vi "FrameParser.vi"(0 "DataIn":u8[](array[numeric]), 1 "frameBuffer":u8[](array[numeric]), 3 "state_in":i32, 4 "dataCnt_in":i32) -> (13 "frameComplete":i32, 14 "frame_data":u8[](array[numeric]), 15 "frame_size":i32, 16 "DataOut":u8[](array[numeric]), 17 "rest":i32, 18 "state_out":i32, 19 "fdataCnt":i32)   [LabVIEW 2017]
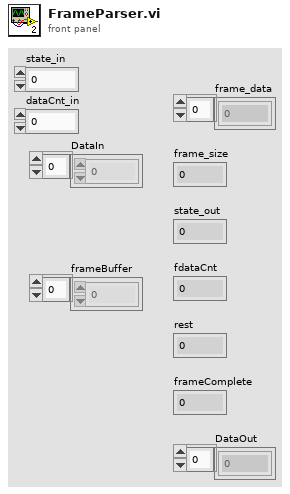
[diagram p1: front panel]
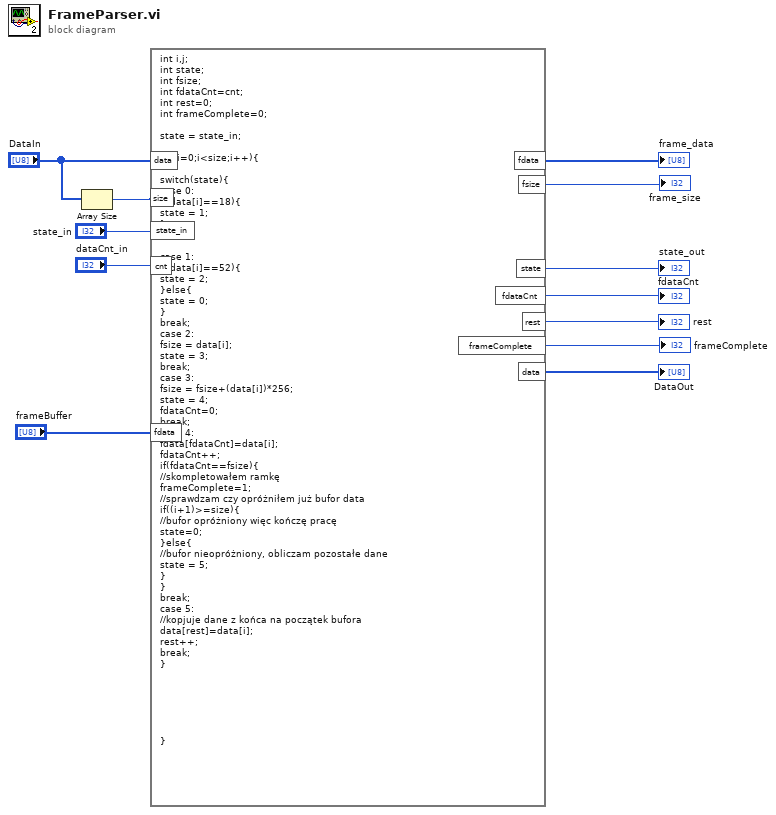
[diagram p0: block diagram]
diagram:
  n1 = Array Size(array="DataIn") -> (size(s)=w3:i32)
  n2 = formula code="int i,j;\nint state;\nint fsize;\nint fdataCnt=cnt;\nint rest=0;\nint frameComplete=0;\n\nstate = state_in;\n\nfor(i=0;i<size;i++){\n\nswitch(state){\ncase 0:\nif(data[i]==18){\nstate = 1;\n}\nbreak;\n\ncase 1:\nif(data[i]==52){\nstate = 2;\n}else{\nstate = 0;\n}\nbreak;\ncase 2:\nfsize = data[i];\nstate = 3;\nbreak;  \ncase 3:\nfsize = fsize+(data[i])*256;\nstate = 4;\nfdataCnt=0;\nbreak;\ncase 4:\nfdata[fdataCnt]=data[i];\nfdataCnt++;\nif(fdataCnt==fsize){\n//skompletowałem ramkę\nframeComplete=1;\n//sprawdzam czy opróżniłem już bufor data\nif((i+1)>=size){\n//bufor opróżniony więc kończę pracę\nstate=0;\n}else{\n//bufor nieopróżniony, obliczam pozostałe dane\nstate = 5;\n}\n}\nbreak;\ncase 5:\n//kopjuje dane z końca na początek bufora\ndata[rest]=data[i];\nrest++;\nbreak;\n}\n\n\n\n\n\n\n}"("data"="DataIn", "size"=w3, "state_in"="state_in", "fdata"="frameBuffer", "cnt"="dataCnt_in") -> ("rest"=→"rest":i32, "fdata"=→"frame_data":u8[], "fsize"=→"frame_size":i32, "state"=→"state_out":i32, "fdataCnt"=→"fdataCnt":i32, "frameComplete"=→"frameComplete":i32, "data"=→"DataOut":u8[])
